vi "main.vi"() -> ()   [LabVIEW 2011]
uses:
  <vilib>/Platform/TimedLoop/XDataNode/timing_clust.ctl
  <vilib>/Platform/TimedLoop/XDataNode/nitl_modes.ctl
  <vilib>/Platform/TimedLoop/XDataNode/wakeup.ctl
  <vilib>/rvi/eio/common/nirviEmuTemplateMethod_errors.vi
  <vilib>/Platform/TimedLoop/XDataNode/XDataNode.xnode
  <vilib>/eio/EIONode/EIONode.xnode
  <vilib>/Platform/TimedLoop/XDataNode/XDNodeRunTimeDep.lvlib
panel:
  in  "Sensor Number":T1(ring)
  out "ticks/count":u32
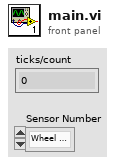
[diagram p1: front panel]
types:
  T1 = enum16{"Wheel Speed 1", "Wheel Speed 2", "Wheel Speed 3", "Wheel Speed 4"}
  T2 = typedef "XDNodeRunTimeDep.lvlib/timing_clust.ctl" = cluster{"Expected End [f-1]":u64, "Actual End [f-1]":u64, "Finished Late? [f-1]":bool, "Expected End [i-1]":u64, "Actual End [i-1]":u64, "Finished Late? [i-1]":bool, "Expected Start [i]":u64, "Actual Start [i]":u64, "Expected Start [f]":u64, "Actual Start [f]":u64, "Source Name":string, "Structure Name":string, "Period":i64, "Deadline":i64, "Offset":i64, "Start":i64, "Priority":i32, "Timeout":i32, "Mode":T3, "Wakeup Reason":T4, "Error":errorcluster, "Source Type":string, "Secondary Source Type":string, "Global End Time":u64, "Global Start Time":u64, "Frame Duration":u64, "Iteration Duration":u64, "Assigned CPU":i32, "I/O Scan Engine Mode":u32}
  T3 = typedef "XDNodeRunTimeDep.lvlib/nitl_modes.ctl" = enum32{"No Change", "Process missed periods, maintain original phase", "Discard missed periods, maintain original phase", "Process missed periods, ignore original phase", "Discard missed periods, ignore original phase"}
  T4 = typedef "XDNodeRunTimeDep.lvlib/wakeup.ctl" = enum32{"Normal", "Aborted", "Asynchronous wakeup", "Timing source error", "Timed loop error", "Timeout"}
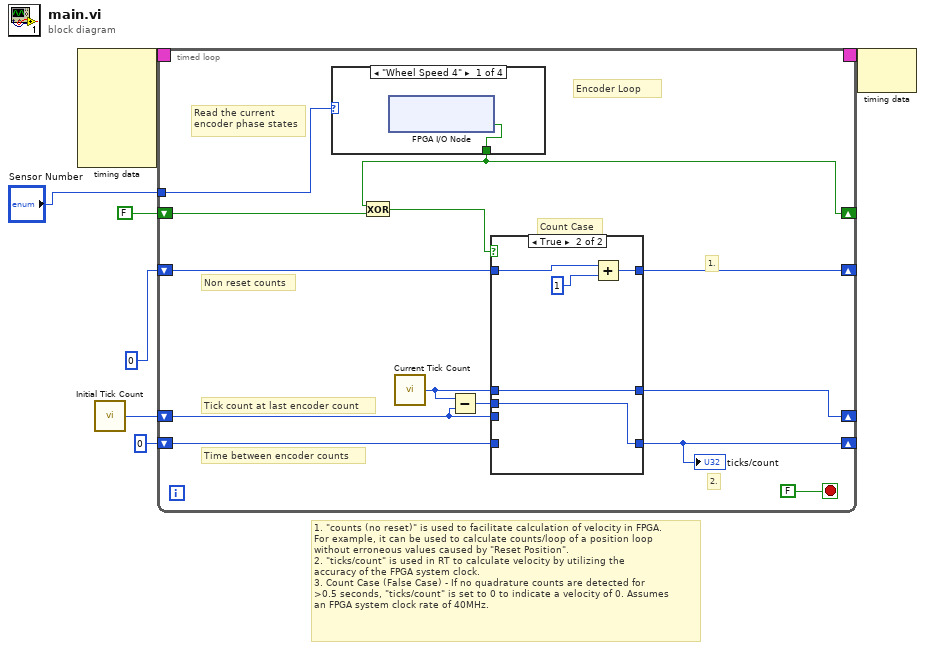
[diagram p0: block diagram]
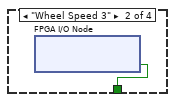
[diagram p2: hidden frame]
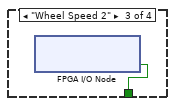
[diagram p3: hidden frame]
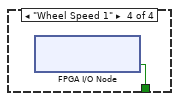
[diagram p4: hidden frame]
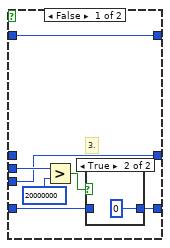
[diagram p5: hidden frame]
diagram:
  # "1. \"counts (no reset)\" is used to facilitate calculation of velocity in FPGA.\nFor example, it can be used to calculate counts/loop of a position loop\nwithout erroneous values caused by \"Reset Position\". \n2. \"ticks/count\" is used in RT to calculate velocity by utilizing the\naccuracy of the FPGA system clock.\n3. Count Case (False Case) - If no quadrature counts are detected for\n>0.5 seconds, \"ticks/count\" is set to 0 to indicate a velocity of 0. Assumes\nan FPGA system clock rate of 40MHz."
  n1 = node-c288() -> (w7:T2)  [unwired: 2 in, 4 out]
  n2 = call "Initial Tick Count"() -> ("Tick Count(Ticks)"=w4:u32)
  n3 = timed-loop {
    shift-right: [w8] -> _
    shift-left: FALSE ("Encoder Phase A") -> [w20]
    shift-right: [w19] -> _
    shift-left: w4 -> [w13]
    shift-right: [w18] -> _
    shift-left: u32 0 -> [w17]
    timing: w7 -> [_]
    timing-out: [_] -> w6
    shift-right: [w14] -> _
    shift-left: 0 ("Reset Position Value") -> [w15]
    tunnel: "Sensor Number" -> [w9]
    stop <- FALSE stop-if-true
    # "Encoder Loop"
    # "Count Case"
    # "2."
    # "1."
    # "Read the current\nencoder phase states"
    # "Non reset counts"
    # "Time between encoder counts"
    # "Tick count at last encoder count"
    n4 = case shown="\"Wheel Speed 4\"" w9 {
      tunnel: [w21 w22 w23 w24] -> w8
      frame "Wheel Speed 4" {
        n5 = xnode "FPGA I/O Node"() -> ("Mod1/DIO4"=w21:bool)  [unwired: 1 in, 1 out]
      }
      frame "Wheel Speed 3" {
        n6 = xnode "FPGA I/O Node"() -> ("Mod1/DIO2"=w22:bool)  [unwired: 1 in, 1 out]
      }
      frame "Wheel Speed 2" {
        n7 = xnode "FPGA I/O Node"() -> ("Mod1/DIO1"=w23:bool)  [unwired: 1 in, 1 out]
      }
      frame "Wheel Speed 1" {
        n8 = xnode "FPGA I/O Node"() -> ("Mod1/DIO0"=w24:bool)  [unwired: 1 in, 1 out]
      }
    }
    n9 = Exclusive Or(1:w20, 2:w8) -> (0:w10:bool)
    n10 = call "Current Tick Count"() -> ("Tick Count(Ticks)"=w11:u32)
    n11 = Subtract(x=w11, y=w13) -> (x-y=w12:u32)
    n12 = case shown="True" w10 {
      tunnel: [w25 w36] -> w19
      tunnel: w13 -> [w25 _]
      tunnel: [w28 w35] -> w18
      tunnel: w17 -> [w27 _]
      tunnel: [w31 w38] -> w14
      tunnel: w15 -> [w31 w37]
      tunnel: w12 -> [w26 w35]
      tunnel: w11 -> [_ w36]
      frame False {
        # "3."
        n13 = Greater?(x=w26, y=20000000 ("x")) -> (0:w29:bool)
        n14 = case shown="True" w29 {
          tunnel: [w32 u32 0] -> w28
          tunnel: w27 -> [w32 _]
          frame False {
          }
          frame True {
          }
        }
      }
      frame True {
        n15 = Add(x=w37, y=1 ("16 bit")) -> (x+y=w38:i32)
      }
    }
    "ticks/count" <- w18
  }
  n16 = node-c288(w6) -> ()  [unwired: 1 out]
